vi "DSF.Engine.Interface.Builder.Write.Command.vi"(6 "overwrite on timeout (T)":bool, 8 "error in (no error)":errorcluster, 9 "timeout in ms (0)":i32 format="%d ms", 10 "command":T3, 11 "Builder Interface in":refnum<class "DSF.Engine.Interface.Builder.lvclass">) -> (0 "error out":errorcluster, 1 "timed out?":bool, 2 "expected response":T1, 3 "Builder Interface out":refnum<class "DSF.Engine.Interface.Builder.lvclass">)   [LabVIEW 2017, in "DSF.Engine.lvlib" / "DSF.Engine.Interface.Builder.lvclass"]
uses:
  DSF.Engine.Interface.Builder.lvclass
  C:/github/data-sharing-framework/dsf core/Source/Engine/Classes/Interface/DSF.Engine.Interface.lvclass
  DSF.Engine.Interface.Builder.Command Data.ctl
  DSF.Engine.Interface.Builder.Command.ctl
  DSF.Engine.Interface.Builder.Response Data.ctl
  DSF.Engine.Interface.Builder.Response.ctl
  DSF.Engine.Interface.lvclass/DSF.Engine.Interface.ctl
  DSF.Engine.Interface.RT FIFO.Data.16B.ctl
  DSF.Engine.Interface.RT FIFO.Payload.16B.ctl
  Debug/DSF.Engine.Debug Flags.FIFO.lvclass/DSF.Engine.Debug Flags.FIFO.ctl
  Debug/DSF.Engine.Debug Flags.FIFO.Get Infinite Timeouts.vi
  Debug/DSF.Engine.Debug Flags.FIFO.lvclass
  DSF.Engine.Interface.lvclass
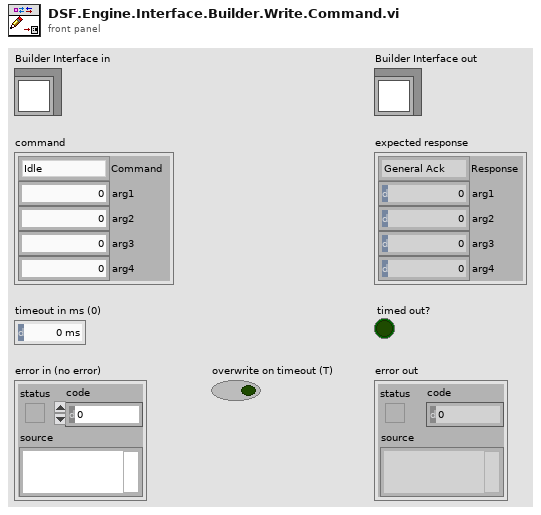
[diagram p1: front panel]
types:
  T1 = typedef "DSF.Engine.lvlib/DSF.Engine.Interface.Builder.lvclass/DSF.Engine.Interface.Builder.Response Data.ctl" = cluster{"Response":T2, "arg1":i32, "arg2":i32, "arg3":i32, "arg4":i32}
  T2 = typedef "DSF.Engine.lvlib/DSF.Engine.Interface.Builder.lvclass/DSF.Engine.Interface.Builder.Response.ctl" = enum8{"General Ack", "Initialize Complete", "Build Complete", "Parse Complete", "Shutdown Ack"}
  T3 = typedef "DSF.Engine.lvlib/DSF.Engine.Interface.Builder.lvclass/DSF.Engine.Interface.Builder.Command Data.ctl" = cluster{"Command":T4, "arg1":i32, "arg2":i32, "arg3":i32, "arg4":i32}
  T4 = typedef "DSF.Engine.lvlib/DSF.Engine.Interface.Builder.lvclass/DSF.Engine.Interface.Builder.Command.ctl" = enum8{"Idle", "Initialize", "Build Buffer", "Parse Buffer", "Shutdown"}
  T5 = typedef "DSF.Engine.lvlib/DSF.Engine.Interface.lvclass/DSF.Engine.Interface.RT FIFO.Data.16B.ctl" = cluster{"Command":u8, "Payload":T6}
  T6 = typedef "DSF.Engine.lvlib/DSF.Engine.Interface.lvclass/DSF.Engine.Interface.RT FIFO.Payload.16B.ctl" = cluster{"arg1":u64, "arg2":u64}
  T7 = typedef "DSF.Engine.lvlib/DSF.Engine.Interface.lvclass/DSF.Engine.Interface.RT FIFO.Ref.16B.ctl" = refnum<k33>
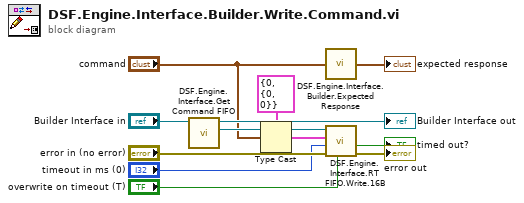
[diagram p0: block diagram]
diagram:
  n1 = call "DSF.Engine.Interface.Get Command FIFO.vi"("Interface in"="Builder Interface in") -> ("Command FIFO"=w12:T7, "Interface out"=→"Builder Interface out":refnum<class "DSF.Engine.Interface.Builder.lvclass">)  [unwired: 9 in]
  n2 = Type Cast(type=T5 {"Command"=0, "Payload"={"arg1"=0, "arg2"=0}} ("element"), x="command") -> (*(type *) &x=w5:T5)
  n3 = call "DSF.Engine.Interface.Builder.Expected Response.vi"("Command"="command") -> ("Response"=→"expected response":T1)
  n4 = call "DSF.Engine.Interface.RT FIFO.Write.16B.vi"("overwrite on timeout (T)"="overwrite on timeout (T)", "error in (no error)"="error in (no error)", "timeout in ms (0)"="timeout in ms (0)", "element"=w5, "RT FIFO in"=w12) -> ("error out"=→"error out":errorcluster, "timed out?"=→"timed out?":bool)  [unwired: 4 in, 1 out]
